vi "Attacker Stop.vi"(6 "atacando contra?":bool, 8 "IA State Input 2":T1, 9 "balls":T4[](array[typedef]), 10 "Field Size in":T5, 11 "Robot in":T2) -> (3 "Robot out":T2)   [LabVIEW 2016]
uses:
  Core/Field Size.ctl
  Core/AI Robot.ctl
  Functions Enum.ctl
  Core/AI Ball.ctl
  Core/AI Input.ctl
  Core/AI Judge.ctl
  Command Enum.ctl
  <vilib>/Analysis/_algsub.llb/Real Vector Norm.vi
  <vilib>/Analysis/NI_AALPro.lvlib
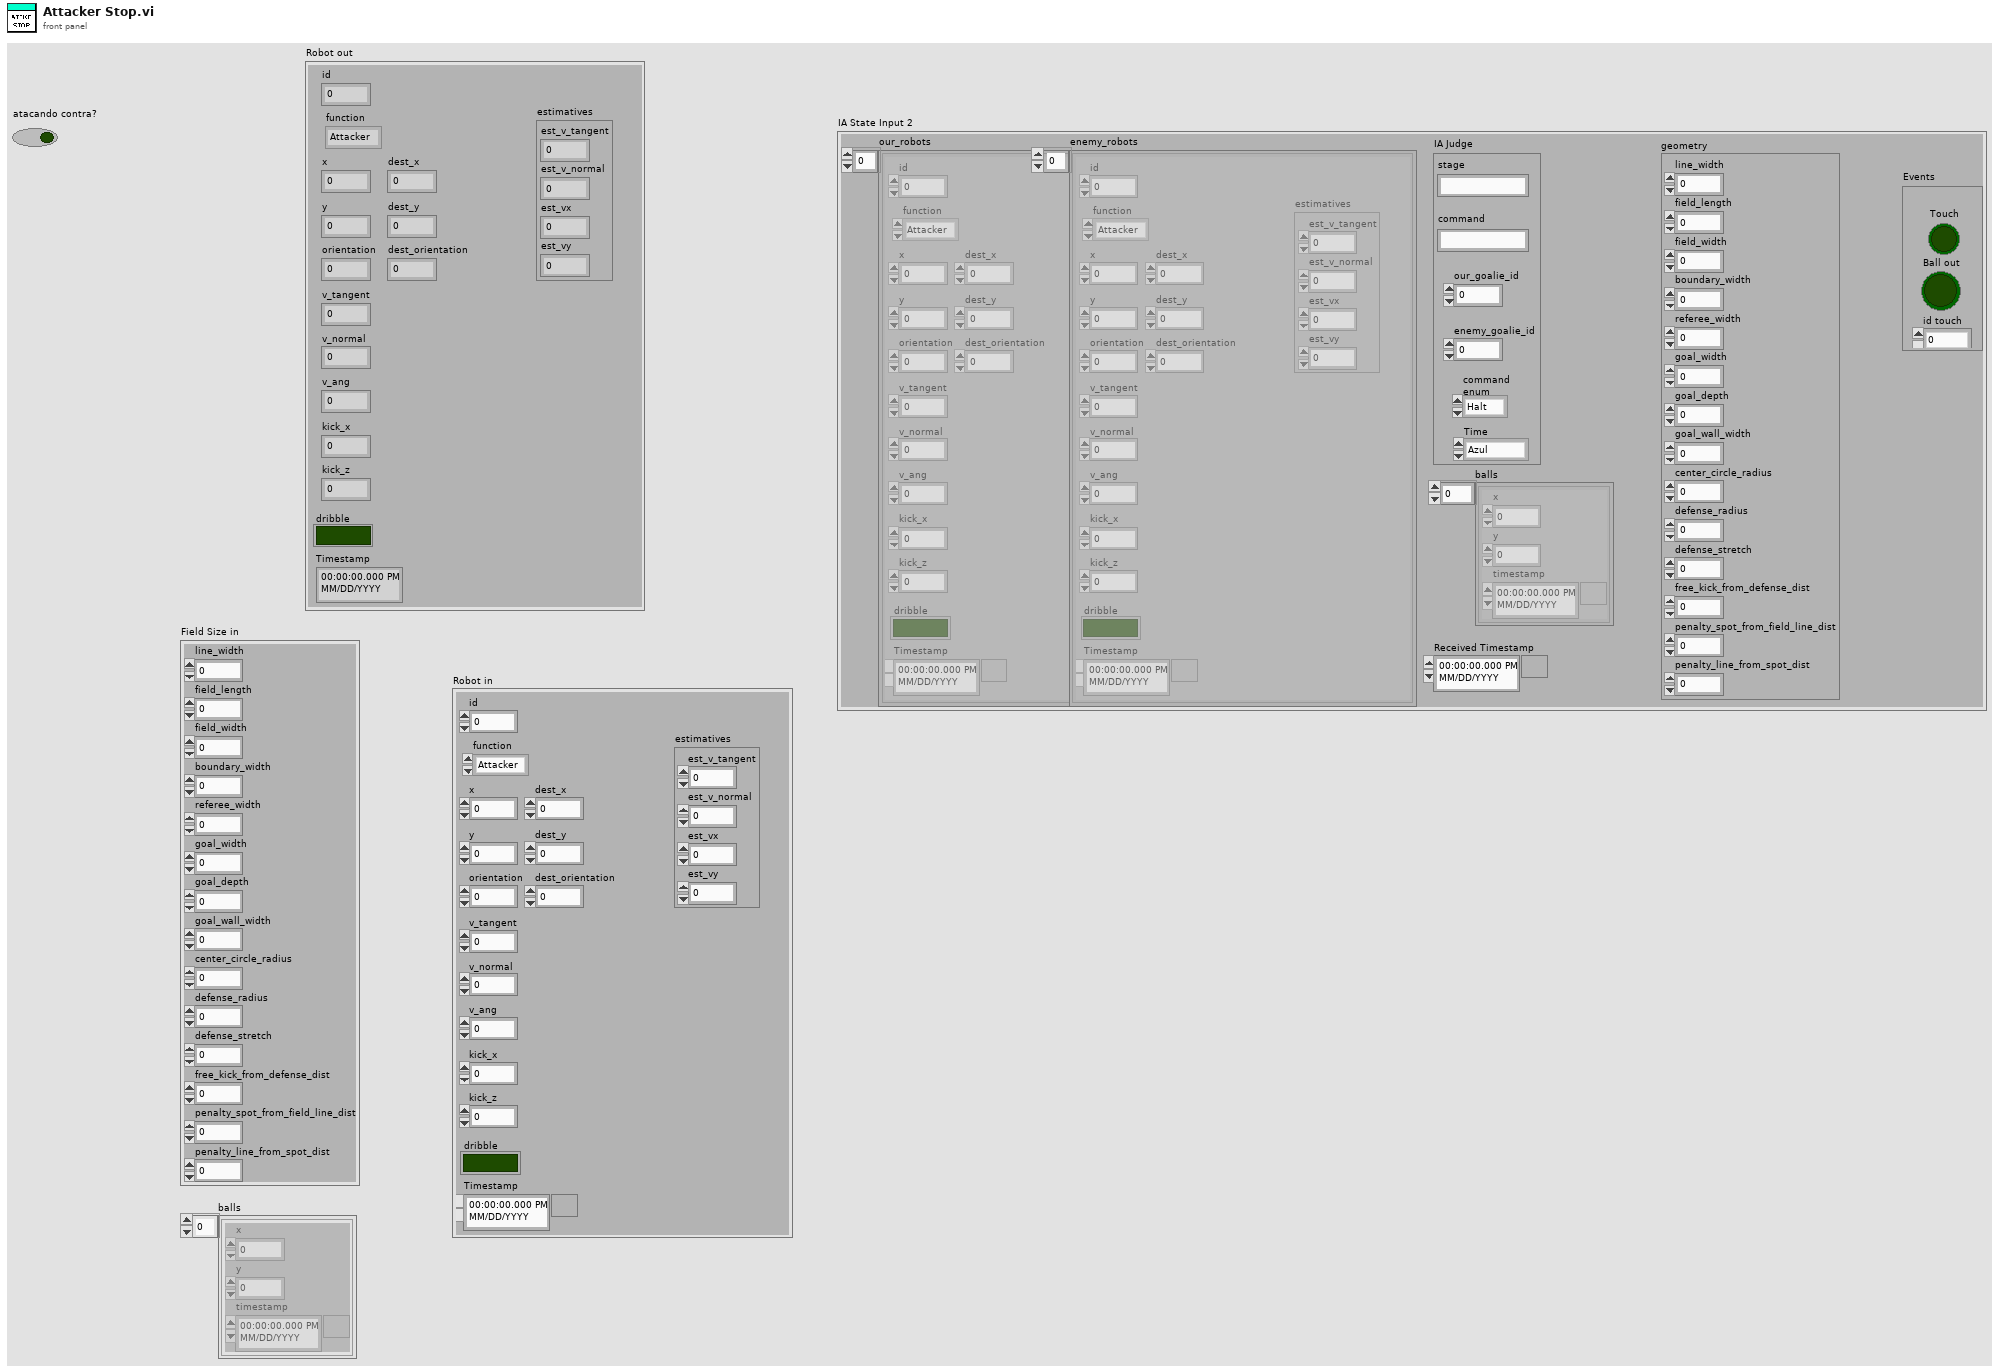
[diagram p1: front panel]
types:
  T1 = typedef "AI Input.ctl" = cluster{"our_robots":T2[], "enemy_robots":T2[], "balls":T4[], "geometry":T5, "IA Judge":T6, "Received Timestamp":timestamp, "Events":cluster{"Touch":bool, "Ball out":bool, "id touch":dbl}}
  T2 = typedef "AI Robot.ctl" = cluster{"id":u32, "function":T3, "x":dbl, "y":dbl, "orientation":dbl, "v_tangent":dbl, "v_normal":dbl, "v_ang":dbl, "kick_x":dbl, "kick_z":dbl, "dribble":bool, "Timestamp":timestamp, "dest_x":dbl, "dest_y":dbl, "dest_orientation":dbl, "estimatives":cluster{"est_v_tangent":dbl, "est_v_normal":dbl, "est_vx":dbl, "est_vy":dbl}}
  T3 = typedef "Functions Enum.ctl" = enum16{"Attacker", "Goalie", "Defender", "Striker", "Goto 0", "Dummy", "ZigZag"}
  T4 = typedef "AI Ball.ctl" = cluster{"x":dbl, "y":dbl, "timestamp":timestamp}
  T5 = typedef "Field Size.ctl" = cluster{"line_width":u32, "field_length":u32, "field_width":u32, "boundary_width":u32, "referee_width":u32, "goal_width":u32, "goal_depth":u32, "goal_wall_width":u32, "center_circle_radius":u32, "defense_radius":u32, "defense_stretch":u32, "free_kick_from_defense_dist":u32, "penalty_spot_from_field_line_dist":u32, "penalty_line_from_spot_dist":u32}
  T6 = typedef "AI Judge.ctl" = cluster{"stage":string, "command":string, "our_goalie_id":dbl, "enemy_goalie_id":dbl, "command\nenum":T7, "Time":enum16{"Azul", "Amarelo"}}
  T7 = typedef "Command Enum.ctl" = enum16{"Halt", "Stop", "Force Start", "PKA Normal Start", "Prepare Kickoff Ally", "PKE Normal Start", "Prepare Kickoff Enemy", "Prepare Penalty Ally", "PPA Normal Start", "Prepare Penalty Enemy", "PPE Normal Start", "Direct Free Enemy", "Direct Free Ally", "Indirect Free Enemy", "Indirect Free Ally", "Timeout Enemy", "Timeout Ally", "Goal Enemy", "Goal Ally", "Ball Placement Enemy", "Ball Placement Ally", "None"}
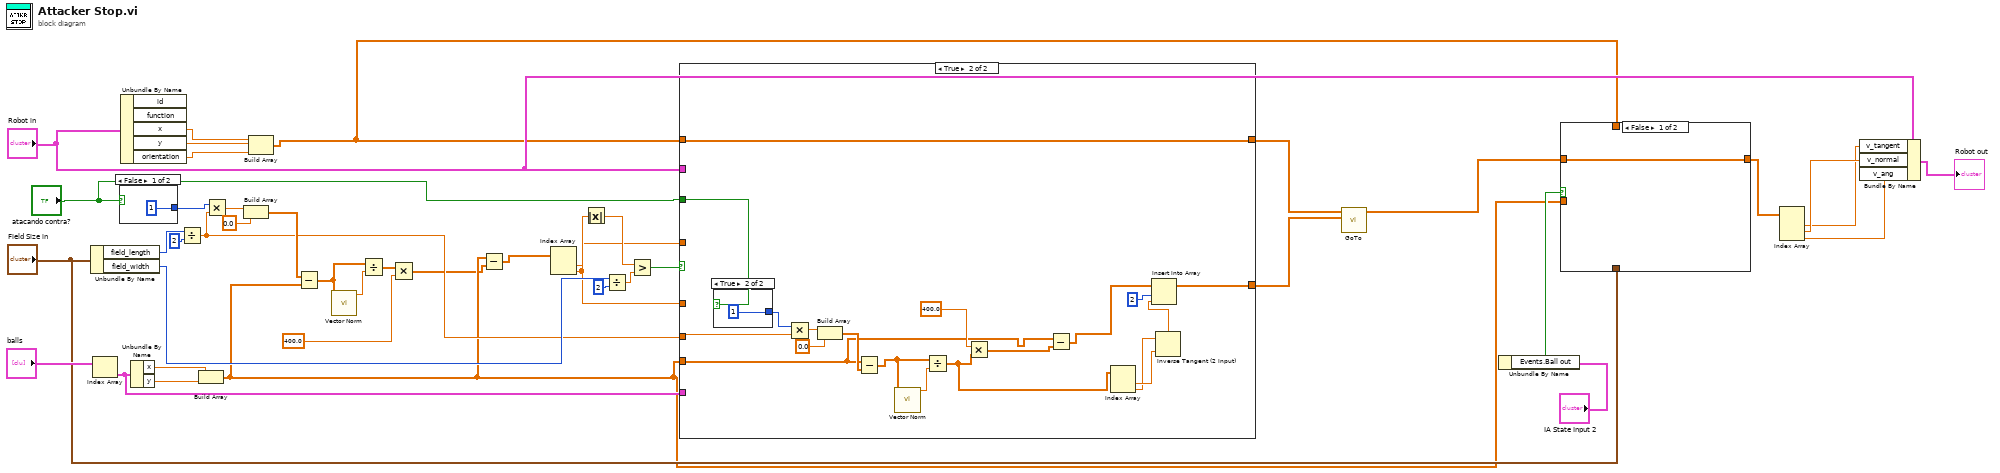
[diagram p0: block diagram]
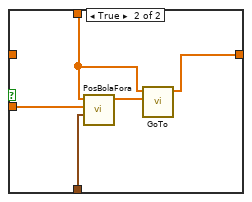
[diagram p2: hidden frame]
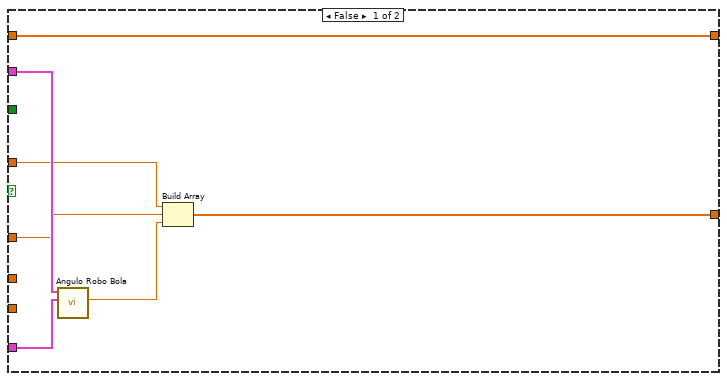
[diagram p3: hidden frame]
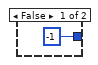
[diagram p4: hidden frame]
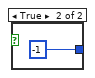
[diagram p5: hidden frame]
diagram:
  n1 = Unbundle By Name("Field Size in") -> ("field_length"=w41:u32, "field_width"=w28:u32)
  n2 = Index Array(array="balls") -> (element=w25:T4)  [unwired: 1 in]
  n3 = case shown="False" "atacando contra?" {
    tunnel: [1 -1] -> w39
    frame False {
    }
    frame True {
    }
  }
  n4 = Unbundle By Name("Robot in") -> ("x"=w21:dbl, "y"=w20:dbl, "orientation"=w19:dbl)  [unwired: 2 out]
  n5 = Unbundle By Name(w25) -> ("x"=w38:dbl, "y"=w37:dbl)
  n6 = Divide(x=w41, y=u32 2) -> (x/y=w17:dbl)
  n7 = Build Array(w38, w37) -> (w3:dbl[])
  n8 = Multiply(x=w39, y=w17) -> (x*y=w36:dbl)
  n9 = Build Array(w36, 0.0 ("element")) -> (w34:dbl[])
  n10 = Build Array(w21, w20, w19) -> (w8:dbl[])
  n11 = Subtract(x=w34, y=w3) -> (x-y=w33:dbl[])
  n12 = call-poly <vilib>:"Vector Norm.vi"("Input Vector"=w33) -> ("norm"=w32:dbl)  [unwired: 9 in, 1 out]
  n13 = Divide(x=w33, y=w32) -> (x/y=w31:dbl[])
  n14 = Multiply(x=w31, y=400.0) -> (x*y=w2:dbl[])
  n15 = Subtract(x=w3, y=w2) -> (x-y=w1:dbl[])
  n16 = Index Array(array=w1) -> (element #1=w22:dbl, element #2=w23:dbl)  [unwired: 2 in]
  n17 = Absolute Value(x=w23) -> (abs(x)=w30:dbl)
  n18 = Divide(x=w28, y=u32 2) -> (x/y=w27:dbl)
  n19 = Greater?(x=w30, y=w27) -> (0:w26:bool)
  n20 = case shown="True" w26 {
    tunnel: w25 -> [w51 _]
    tunnel: "Robot in" -> [w50 _]
    tunnel: w23 -> [w48 _]
    tunnel: w22 -> [w47 _]
    tunnel: w8 -> [w46 w57]
    tunnel: w3 -> [_ w53]
    tunnel: "atacando contra?" -> [_ w64]
    tunnel: w17 -> [_ w69]
    tunnel: [w46 w57] -> w6
    tunnel: [w45 w56] -> w5
    frame False {
      n21 = call "Angulo Robo Bola.vi"("Ball"=w51, "Robot"=w50) -> ("Angulo"=w49:dbl)  [unwired: 9 in]
      n22 = Build Array(w47, w48, w49) -> (w45:dbl[])
    }
    frame True {
      n23 = case shown="True" w64 {
        tunnel: [-1 1] -> w70
        frame False {
        }
        frame True {
        }
      }
      n24 = Multiply(x=w70, y=w69) -> (x*y=w68:dbl)
      n25 = Build Array(w68, 0.0 ("element")) -> (w63:dbl[])
      n26 = Subtract(x=w53, y=w63) -> (x-y=w65:dbl[])
      n27 = call-poly <vilib>:"Vector Norm.vi"("Input Vector"=w65) -> ("norm"=w66:dbl)  [unwired: 9 in, 1 out]
      n28 = Divide(x=w65, y=w66) -> (x/y=w58:dbl[])
      n29 = Multiply(x=400.0, y=w58) -> (x*y=w54:dbl[])
      n30 = Subtract(x=w53, y=w54) -> (x-y=w52:dbl[])
      n31 = Index Array(array=w58) -> (element #1=w60:dbl, element #2=w59:dbl)  [unwired: 2 in]
      n32 = Inverse Tangent (2 Input)(1:w60, 2:w59) -> (0:w61:dbl)
      n33 = Insert Into Array(array=w52, index=2, new element=w61) -> (w56:dbl[])
    }
  }
  n34 = call "GoTo.vi"("Target"=w5, "Position"=w6) -> ("Output\nVelocity"=w7:dbl[])  [unwired: 8 in, 1 out]
  n35 = Unbundle By Name("IA State Input 2") -> ("Events.Ball out"=w16:bool)
  n36 = case shown="False" w16 {
    tunnel: w7 -> [w73 _]
    tunnel: [w73 w74] -> w10
    tunnel: "Field Size in" -> [_ w78]
    tunnel: w8 -> [_ w75]
    tunnel: w3 -> [_ w77]
    frame False {
    }
    frame True {
      n37 = call "PosBolaFora.vi"("Field Size in"=w78, "Position da bola"=w77, "Position do robot"=w75) -> ("Target"=w76:dbl[])  [unwired: 8 in]
      n38 = call "GoTo.vi"("Target"=w76, "Position"=w75) -> ("Output\nVelocity"=w74:dbl[])  [unwired: 8 in, 1 out]
    }
  }
  n39 = Index Array(array=w10) -> (element #1=w13:dbl, element #2=w14:dbl, element #3=w15:dbl)  [unwired: 3 in]
  n40 = Bundle By Name(cluster="Robot in", "v_tangent"=w13, "v_normal"=w14, "v_ang"=w15) -> (→"Robot out":T2)
